vi "Save Cp snapshot.vi"(0 "Pdyn ref (Pa)":sgl, 1 "rho ref (kg/m^3)":sgl, 2 "chord (m)":sgl=0.314309, 3 "span (m)":sgl=1.0, 4 "Fx (N)":sgl, 5 "Fy (N)":sgl, 6 "Cp distribution (time averaged)":cluster{"x/c flap (sorted)":sgl[], sgl[]}[](graph), 8 "d.p":i16=4, 10 "File Path":path=path "C:/Datalogs/Cp snapshot 001.txt") -> (19 "error out":errorcluster)   [LabVIEW 2015]
uses:
  <vilib>/Utility/file.llb/Write Delimited Spreadsheet (string).vi
panel:
  in  "y/c flap":sgl[](array[numeric])=[0.3702977, 0.27414677, 0.19456363, 0.14230296, 0.12718599, 0.15663312, 0.19359294, 0.247963]
  in  "y/c wing":sgl[](array[numeric])=[-0.055548523, -0.12028768, -0.124059446, -0.11144002, -0.08997261, -0.06635858, -0.048627622, -0.043094855, -0.034690067, -0.022772176, -0.001057558, 0.02325355, 0.025220403, 0.02517618, 0.023960816, 0.020169007, 0.01457642, -0.00389553, -0.028557567, -0.043236114, -0.04890474, -0.03931195]
  # "Paste in values from Geometry Prep vi"
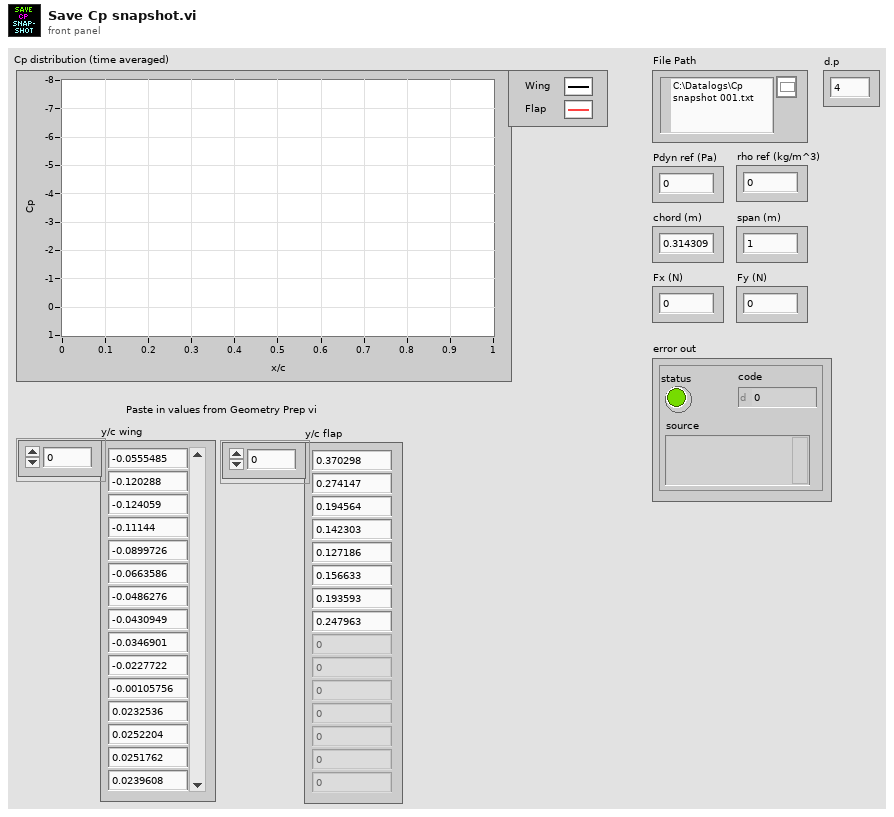
[diagram p1: front panel]
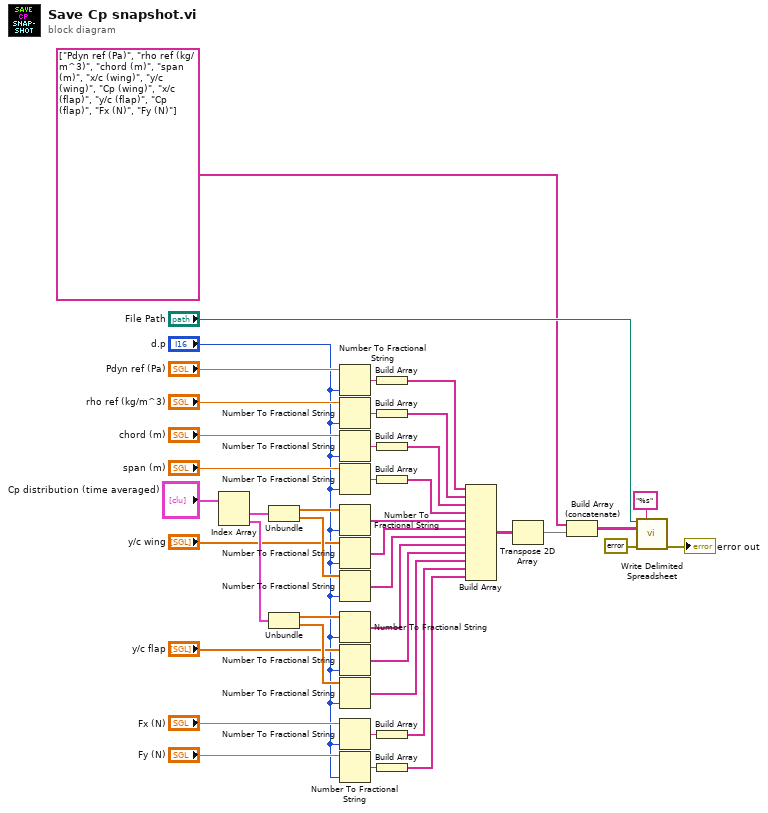
[diagram p0: block diagram]
diagram:
  n1 = Index Array(array="Cp distribution (time averaged)") -> (element #1=w41:cluster{"x/c flap (sorted)":sgl[], sgl[]}, element #2=w40:cluster{"x/c flap (sorted)":sgl[], sgl[]})  [unwired: 2 in]
  n2 = Unbundle(w41) -> ("x/c flap (sorted)"=w39:sgl[], w38:sgl[])
  n3 = Unbundle(w40) -> ("x/c flap (sorted)"=w37:sgl[], w36:sgl[])
  n4 = Number To Fractional String(number="Pdyn ref (Pa)", precision (6)="d.p") -> (F-format string=w24:string)  [unwired: 2 in]
  n5 = Number To Fractional String(number="rho ref (kg/m^3)", precision (6)="d.p") -> (F-format string=w16:string)  [unwired: 2 in]
  n6 = Number To Fractional String(number="chord (m)", precision (6)="d.p") -> (F-format string=w11:string)  [unwired: 2 in]
  n7 = Number To Fractional String(number="span (m)", precision (6)="d.p") -> (F-format string=w10:string)  [unwired: 2 in]
  n8 = Number To Fractional String(number=w39, precision (6)="d.p") -> (F-format string=w35:string[])  [unwired: 2 in]
  n9 = Number To Fractional String(number="y/c wing", precision (6)="d.p") -> (F-format string=w4:string[])  [unwired: 2 in]
  n10 = Number To Fractional String(number=w38, precision (6)="d.p") -> (F-format string=w5:string[])  [unwired: 2 in]
  n11 = Number To Fractional String(number=w37, precision (6)="d.p") -> (F-format string=w34:string[])  [unwired: 2 in]
  n12 = Number To Fractional String(number="y/c flap", precision (6)="d.p") -> (F-format string=w2:string[])  [unwired: 2 in]
  n13 = Number To Fractional String(number=w36, precision (6)="d.p") -> (F-format string=w3:string[])  [unwired: 2 in]
  n14 = Number To Fractional String(number="Fx (N)", precision (6)="d.p") -> (F-format string=w21:string)  [unwired: 2 in]
  n15 = Number To Fractional String(number="Fy (N)", precision (6)="d.p") -> (F-format string=w20:string)  [unwired: 2 in]
  n16 = Build Array(w24) -> (w15:string[])
  n17 = Build Array(w16) -> (w14:string[])
  n18 = Build Array(w11) -> (w9:string[])
  n19 = Build Array(w10) -> (w8:string[])
  n20 = Build Array(w21) -> (w19:string[])
  n21 = Build Array(w20) -> (w18:string[])
  n22 = Build Array(w15, w14, w9, w8, w35, w4, w5, w34, w2, w3, w19, w18) -> (w33:string[][])
  n23 = Transpose 2D Array(2D array=w33) -> (transposed array=w32:string[][])
  n24 = Build Array (concatenate)(string[] ["Pdyn ref (Pa)", "rho ref (kg/m^3)", "chord (m)", "span (m)", "x/c (wing)", "y/c (wing)", "Cp (wing)", "x/c (flap)", "y/c (flap)", "Cp (flap)", "Fx (N)", "Fy (N)"], w32) -> (w31:string[][])
  n25 = call-poly <vilib>:"Write Delimited Spreadsheet.vi"("file path (dialog if empty)"="File Path", "format (%s)"="%s", "2D data"=w31, "error in (no error)"=errorcluster {"status"=FALSE, "code"=0, "source"=""}) -> ("error out"=→"error out":errorcluster)  [unwired: 10 in, 1 out]
